vi "PH_PP_CurrentMeas.ProcEvents.vi"(0 "i ref in":refnum<vi>, 5 "error in":errorcluster) -> (14 "i ref out":refnum<vi>, 19 "error out":errorcluster)   [LabVIEW 2014, in "PH_PP_CurrentMeas.lvlib"]
doc: "This method is used to define the events the object will listen to. Add your own events here."
uses:
  PH_PP_CurrentMeas.lvlib
  CSCore/BaseProcess/BaseProcess.event definition.ctl
  CSCore/CAEObj/CAEObj.event definition.ctl
  CSCore/BaseProcess/BaseProcess.descriptor string definition.ctl
  CSCore/BaseProcess/BaseProcess.lvlib
  CSCore/CAEObj/CAEObj.lvlib
  PH_Common/PH_Common.lvlib
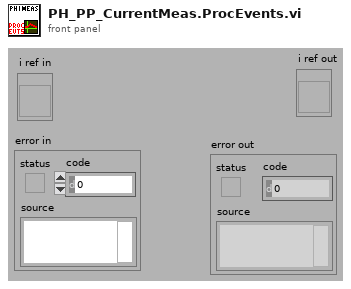
[diagram p1: front panel]
types:
  T1 = typedef "BaseProcess.lvlib/BaseProcess.event definition.ctl" = cluster{"CAEEvtDef":T2, "Data Descriptor":T3}
  T2 = typedef "CAEObj.lvlib/CAEObj.event definition.ctl" = cluster{"URL":string, "enable":bool, "ignoreResID":bool}
  T3 = typedef "BaseProcess.lvlib/BaseProcess.descriptor string definition.ctl" = string
  T4 = typedef "PH_PP_CurrentMeas.lvlib/PH_PP_CurrentMeas.i attribute.ctl" = cluster{"Status":cluster{"GUI Ref Hardware Feedback":refnum<vi>, "Tab Control":refnum<vi>}, "PU 1":cluster{"Instance":string, "Status":T5, "Ref Status ":refnum<vi>, "Data":waveform(dbl)[], "Ref Data":refnum<vi>}, "PU 2":cluster{"Instance":string, "Status":T5, "Ref Status ":refnum<vi>, "Data":waveform(dbl)[], "Ref Data":refnum<vi>}, "PU 3":cluster{"Instance":string, "Status":T5, "Ref Status ":refnum<vi>, "Data":waveform(dbl)[], "Ref Data":refnum<vi>}, "PU 4":cluster{"Instance":string, "Status":T5, "Ref Status ":refnum<vi>, "Data":waveform(dbl)[], "Ref Data":refnum<vi>}, "PU 5":cluster{"Instance":string, "Status":T5, "Ref Status ":refnum<vi>, "Data":waveform(dbl)[], "Ref Data":refnum<vi>}, "FR":cluster{"Instance":string, "Status":T5, "Ref Status ":refnum<vi>, "Data":waveform(dbl)[], "Ref Data":refnum<vi>}, "PA - 19mm 1":cluster{"Instance":string, "Status":T5, "Ref Status ":refnum<vi>}, "PA - 19mm 2":cluster{"Instance":string, "Status":T5, "Ref Status ":refnum<vi>, "no link":bool}, "PA - 45mm":cluster{"Instance":string, "Status":T5, "Ref Status ":refnum<vi>, "no link":bool}, "PA Data":cluster{"Data":waveform(dbl)[], "Ref":refnum<vi>}, "Sequencer":cluster{"Instance":string, "SM State Ref":refnum<vi>}, "Tasks":cluster{"Port":u16, "connection ID":refnum<k5>, "Status":T5, "Ref":refnum<vi>, "Ref Bar":refnum<vi>, "Feedback":cluster{"Received Data Sets":T6[], "Driver Error":errorcluster, "Connection not established":bool, "Error unpacking the data":bool, "No Task defined":bool, "Not triggered yet":bool}, "Data":waveform(dbl)[], "Ref Teststart Task":refnum<vi>}[], "in use":cluster{"MA DP":bool, "FR and PA":bool}, "DAQ Server":string}
  T5 = typedef "PH_StatusHandler.lvlib/PH_StatusHandler.Status.ctl" = i16
  T6 = typedef "PH_PP_CurrentMeas.lvlib/PH_PP_CurrentMeas.CommandCluster.ctl" = cluster{"Command":string, "Data":string, "error out":errorcluster}
  T7 = typedef "PH_Common.lvlib/PH_DIM.Event Declarer.ctl" = cluster{"Service Name":string, "Selector":string}
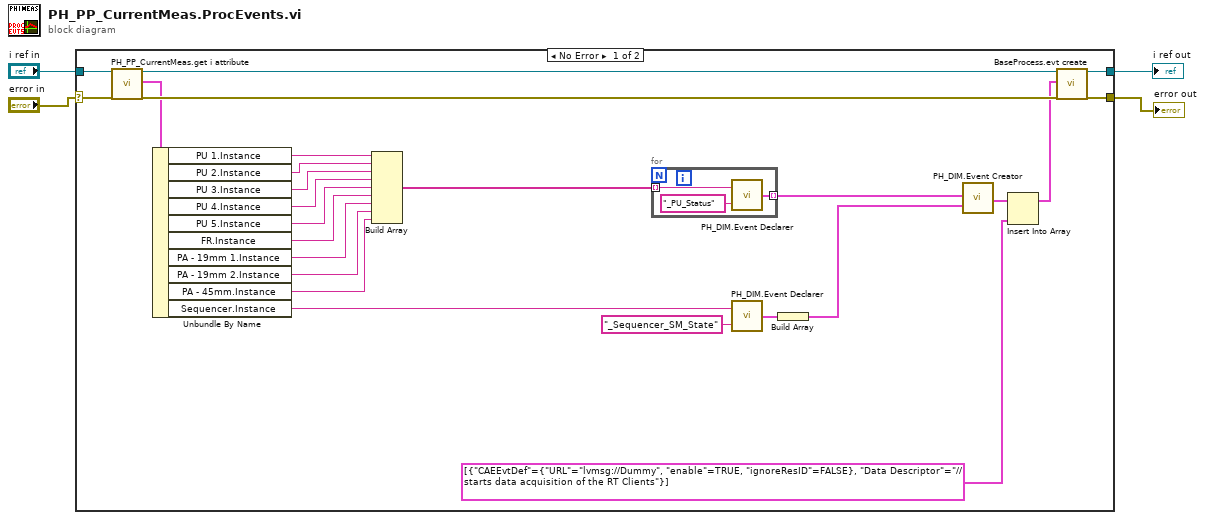
[diagram p0: block diagram]
diagram:
  n1 = case shown="No Error" "error in" {
    selector: "error in" -> [w25 w33]
    tunnel: "i ref in" -> [w27 w34]
    tunnel: [w29 w34] -> w3
    tunnel: [w28 w33] -> w2
    frame No Error {
      n2 = call "PH_PP_CurrentMeas.get i attribute.vi"("i ref in"=w27, "error in (no error)"=w25) -> ("i ref out"=w26:refnum<vi>, "i attribute"=w23:T4, "error out"=w24:errorcluster)  [unwired: 15 in]
      n3 = Unbundle By Name(w23) -> ("PU 1.Instance"=w18:string, "PU 2.Instance"=w16:string, "PU 3.Instance"=w15:string, "PU 4.Instance"=w14:string, "PU 5.Instance"=w13:string, "FR.Instance"=w12:string, "PA - 19mm 1.Instance"=w11:string, "PA - 19mm 2.Instance"=w10:string, "PA - 45mm.Instance"=w9:string, "Sequencer.Instance"=w8:string)
      n4 = Build Array(w18, w16, w15, w14, w13, w12, w11, w10, w9) -> (w17:string[])
      n5 = for {
        tunnel: [w31] -> w19 mode=indexing
        tunnel: w17 -> [w32] mode=indexing
        n6 = call "PH_DIM.Event Declarer.vi"("Selector"="_PU_Status" ("URL"), "Service Name"=w32) -> ("declared DIM Event"=w31:T7)
      }
      n7 = call "PH_DIM.Event Declarer.vi"("Selector"="_Sequencer_SM_State", "Service Name"=w8) -> ("declared DIM Event"=w6:T7)
      n8 = Build Array(w6) -> (w5:T7[])
      n9 = call "PH_DIM.Event Creator.vi"("Status Services"=w19, "SM State Services"=w5) -> ("DIM Service Events"=w21:T1[])  [unwired: 17 in]
      n10 = Insert Into Array(array=w21, new element=T1[] [{"CAEEvtDef"={"URL"="lvmsg://Dummy", "enable"=TRUE, "ignoreResID"=FALSE}, "Data Descriptor"="//starts data acquisition of the RT Clients"}] ("new events(V3.0)")) -> (w22:T1[])  [unwired: 1 in]
      n11 = call "BaseProcess.evt create.vi"("i ref in"=w26, "newEvents"=w22, "error in (no error)"=w24) -> ("i ref out"=w29:refnum<vi>, "error out"=w28:errorcluster)  [unwired: 13 in, 2 out]
    }
    frame Error {
    }
  }
  "i ref out" <- w3
  "error out" <- w2
